vi "Error Handler - Message Handling Loop.vi"(8 "error in (no error)":cluster{"状态":bool, "代码":i32, "源":string} caption="错误输入（无错误）", 10 "忽略错误（运行时）":i32[](array[numeric]), 11 "消息队列":refnum<queue>) -> (0 "错误输入副本":cluster{"状态":bool, "代码":i32, "源":string}, 3 "消息队列副本":refnum<queue>)   [LabVIEW 2025]
doc: "对“消息处理循环”中出现的错误进行处理：忽略该错误，或者为该错误生成一个“退出”(Exit)消息。"
uses:
  Message Queue/Message Cluster.ctl
  Message Queue/Message Queue.lvlib
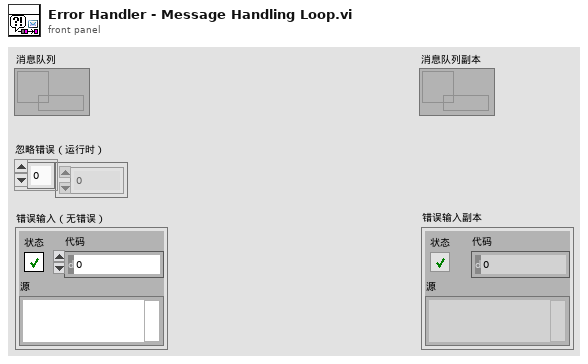
[diagram p1: front panel]
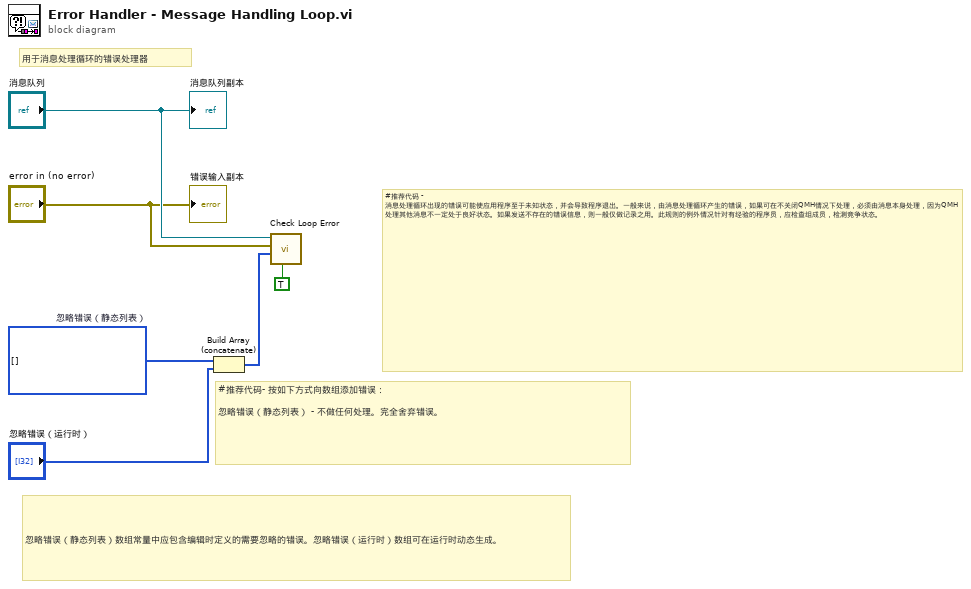
[diagram p0: block diagram]
diagram:
  w5 = i32[] []  # 忽略错误（静态列表）
  # "#推荐代码 - 消息处理循环出现的错误可能使应用程序至于未知状态，并会导致程序退出。一般来说，由消息处理循环产生的错误，如果可在不关闭QMH情况下处理，必须由消息本身处理，因为QMH处理其他消息不一定处于良好状态。如果发送不存在的错误信息，则一般仅做记录之用。此规则的例外情况针对有经验的程序员，应检查组成员，检测竞争状态。"
  # "忽略错误（静态列表）数组常量中应包含编辑时定义的需要忽略的错误。忽略错误（运行时）数组可在运行时动态生成。"
  # "#推荐代码- 按如下方式向数组添加错误：\n\n忽略错误（静态列表） - 不做任何处理。完全舍弃错误。"
  # "用于消息处理循环的错误处理器"
  n1 = Build Array (concatenate)(w5, "忽略错误（运行时）") -> (w4:i32[])
  n2 = call "Check Loop Error.vi"("错误时退出？ (F)"=TRUE ("Exit on Error? (F)"), "忽略错误"=w4, "待处理的错误"="error in (no error)", "消息队列"="消息队列") -> ()  [unwired: 6 in, 2 out]
  "消息队列副本" <- "消息队列"
  "错误输入副本" <- "error in (no error)"
